vi "Wait on State.vi"(8 "error in (no error)":errorcluster, 9 "Timeout ms (-1)":i32=-1, 10 "State":T1, 11 "Connection in":refnum<class "Connection.lvclass">) -> (0 "error out":errorcluster, 1 "Timed Out?":bool, 3 "Connection out":refnum<class "Connection.lvclass">)   [LabVIEW 2020, in "Stream.lvlib" / "Connection.lvclass"]
uses:
  Connection.lvclass
  State.ctl
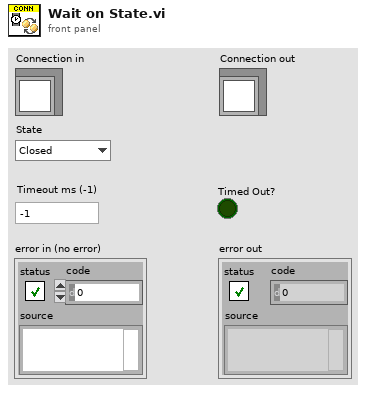
[diagram p1: front panel]
types:
  T1 = typedef "Stream.lvlib/Connection.lvclass/State.ctl" = enum16{"Closed", "Idle", "Connecting", "Connected", "Shutdown"}
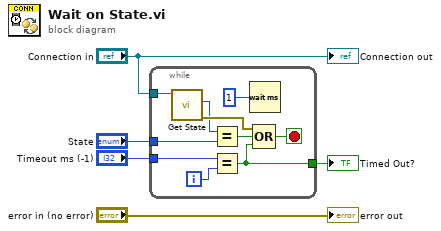
[diagram p0: block diagram]
diagram:
  n1 = while {
    tunnel: "Connection in" -> [w15]
    tunnel: "State" -> [w12]
    tunnel: "Timeout ms (-1)" -> [w10]
    tunnel: [w7] -> w1
    i -> [w9]
    stop <- w8 stop-if-true
    n2 = call "Get State.vi"("Connection in"=w15) -> ("error out"=w14:errorcluster, "State"=w13:T1)  [unwired: 8 in, 1 out]
    n3 = Equal?(x=w13, y=w12) -> (x = y?=w11:bool)
    n4 = Equal?(x=w10, y=w9) -> (x = y?=w7:bool)
    n5 = Wait (ms)(milliseconds to wait=u32 1) -> ()  [unwired: 1 out]
    n6 = Compound Arithmetic op=OR(w14, w11, w7) -> (w8:bool)
  }
  "Timed Out?" <- w1
  "error out" <- "error in (no error)"
  "Connection out" <- "Connection in"
